vi "from string.vi"(8 "error in":errorcluster, 9 "data":string, 10 "version":string, 11 "fixed channel configuration in":refnum<class "control module configuration.lvclass">) -> (0 "error out":errorcluster, 3 "fixed channel configuration out":refnum<class "control module configuration.lvclass">)   [LabVIEW 2013, in "control module configuration.lvclass"]
doc: "Provides an interface for loading a module configuration from a file or other serialized data source. It is recommended that all children of this class store data in two sets--data required for its own initialization, and any data required for parent initialization--and that each implementation uses the <b>Call Parent Method</b> primitive to de-serialize parent information. As a result, it is expected that every module configuration class calls <b>component configuration.lvclass:From String.vi</b>.\nNI Tag Bus Module Framework 1.0.3.43\nNI Systems Engineering"
uses:
  control module configuration.lvclass
  <vilib>/NI/Tag Bus Module Framework/module configuration/TBM module configuration.lvclass
  <vilib>/NI/Tag Bus Module Framework/channel/TBM channel.lvclass
  control module configuration.lvclass/control module configuration.ctl
  <vilib>/NI/Configuration Framework/serializable configuration/NISE_CEF_serializable configuration.lvclass
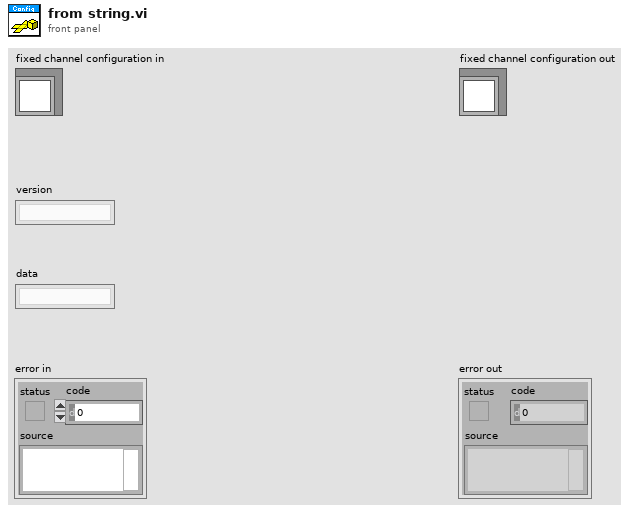
[diagram p1: front panel]
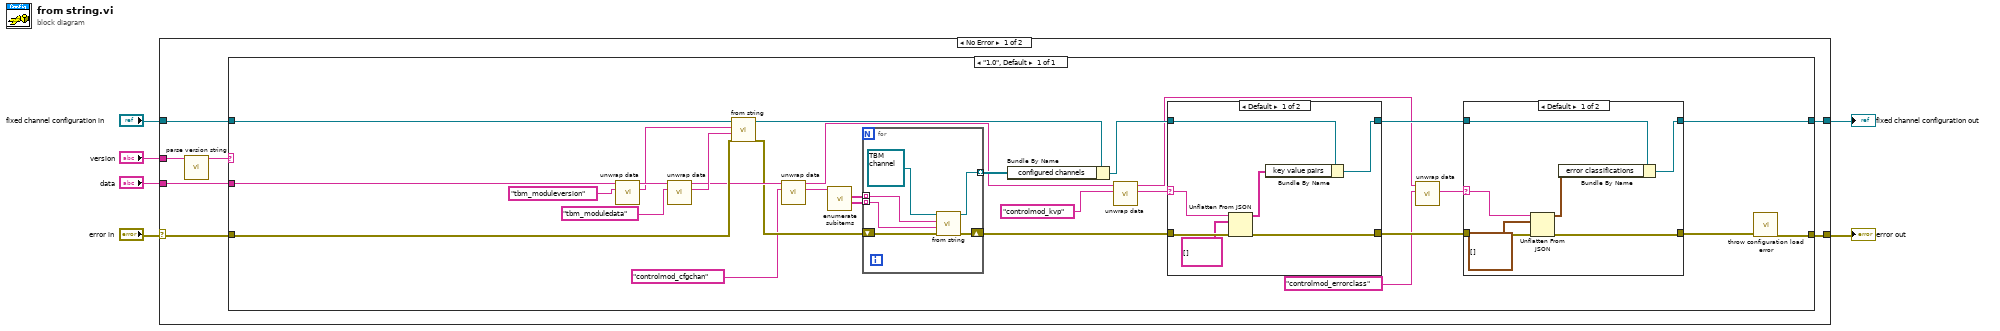
[diagram p0: block diagram]
diagram:
  n1 = case shown="No Error" "error in" {
    selector: "error in" -> [w7 w68]
    tunnel: "data" -> [w13 _]
    tunnel: "fixed channel configuration in" -> [w12 w67]
    tunnel: [w11 w67] -> w5
    tunnel: [w10 w68] -> w4
    tunnel: "version" -> [w9 _]
    frame No Error {
      n2 = call <vilib>:"parse version string.vi"("full version"=w9) -> ("major.minor version"=w8:string)  [unwired: 7 in, 3 out]
      n3 = case shown="\"1.0\", Default" w8 {
        tunnel: w13 -> [w38]
        tunnel: w7 -> [w40]
        tunnel: w12 -> [w42]
        tunnel: [w39] -> w11
        tunnel: [w41] -> w10
        frame "1.0", Default {
          n4 = call <vilib>:"unwrap data.vi"("identifier"="tbm_moduleversion" ("additional identifier"), "data to unwrap"=w38) -> ("unwrapped data"=w32:string, "remaining string"=w34:string)  [unwired: 8 in]
          n5 = call <vilib>:"unwrap data.vi"("identifier"="tbm_moduledata" ("additional identifier"), "data to unwrap"=w34) -> ("unwrapped data"=w33:string, "remaining string"=w31:string)  [unwired: 8 in]
          n6 = call-parent "from string.vi"("error in"=w40, "data"=w33, "version"=w32, "module configuration in"=w42) -> ("error out"=w29:errorcluster, "module configuration out"=w37:refnum<class "control module configuration.lvclass">)  [unwired: 6 in]
          n7 = call <vilib>:"unwrap data.vi"("identifier"="controlmod_cfgchan", "data to unwrap"=w31) -> ("unwrapped data"=w30:string, "remaining string"=w25:string)  [unwired: 8 in]
          n8 = call <vilib>:"enumerate subitems.vi"("data to enumerate"=w30) -> ("associated data"=w27:string[], "discovered subitems"=w28:string[])  [unwired: 8 in, 1 out]
          n9 = for {
            shift-right: [w66] -> w24
            shift-left: w29 -> [w65]
            tunnel: w28 -> [w63] mode=indexing
            tunnel: w27 -> [w62] mode=indexing
            tunnel: [w64] -> w26 mode=indexing
            n10 = call-dynamic "from string.vi"("error in"=w65, "channel data"=w62, "identifier"=w63, "channel in"=refnum<class "TBM channel.lvclass"> refnum) -> ("error out"=w66:errorcluster, "channel out"=w64:refnum<class "TBM channel.lvclass">)  [unwired: 6 in]
          }
          n11 = Bundle By Name(cluster=w37, "configured channels"=w26) -> (w22:refnum<class "control module configuration.lvclass">)
          n12 = call <vilib>:"unwrap data.vi"("identifier"="controlmod_kvp", "data to unwrap"=w25) -> ("unwrapped data"=w23:string, "remaining string"=w17:string)  [unwired: 8 in]
          n13 = case shown="Default" w23 {
            selector: w23 -> [w54 _]
            tunnel: w24 -> [w56 w60]
            tunnel: [w55 w60] -> w21
            tunnel: w22 -> [w58 w59]
            tunnel: [w57 w59] -> w19
            frame Default {
              n14 = Unflatten From JSON(JSON string=w54, type and defaults=string[][] [] ("key value pairs"), error in (no error)=w56) -> (value=w53:string[][], error out=w55:errorcluster)  [unwired: 4 in]
              n15 = Bundle By Name(cluster=w58, "key value pairs"=w53) -> (w57:refnum<class "control module configuration.lvclass">)
            }
            frame "" {
            }
          }
          n16 = call <vilib>:"unwrap data.vi"("identifier"="controlmod_errorclass", "data to unwrap"=w17) -> ("unwrapped data"=w18:string)  [unwired: 8 in, 1 out]
          n17 = case shown="Default" w18 {
            selector: w18 -> [w45 _]
            tunnel: w21 -> [w47 w51]
            tunnel: [w46 w51] -> w20
            tunnel: w19 -> [w49 w50]
            tunnel: [w48 w50] -> w39
            frame Default {
              n18 = Unflatten From JSON(JSON string=w45, type and defaults=cluster{i32, i32}[] [], error in (no error)=w47) -> (value=w44:cluster{i32, i32}[], error out=w46:errorcluster)  [unwired: 4 in]
              n19 = Bundle By Name(cluster=w49, "error classifications"=w44) -> (w48:refnum<class "control module configuration.lvclass">)
            }
            frame "" {
            }
          }
          n20 = call <vilib>:"throw configuration load error.vi"("error in"=w20) -> ("error out"=w41:errorcluster)  [unwired: 10 in]
        }
      }
    }
    frame Error {
    }
  }
  "error out" <- w4
  "fixed channel configuration out" <- w5
